vi "Q8381 REF LEVEL_AUTO.vi"(1 "off/on":sgl(ring) items=["OFF", "ON"], 2 "GPIB Sddress":u16=8 max=31 step=1, 3 "VISA resource name":refnum<visa-resource-name>) -> (0 "GPIB Status":bool)   [LabVIEW 2017]
doc: "off/on: 0: off, 1: on."
panel:
  out "Program Code":string
  # "REF  LEVEL__AUTO"
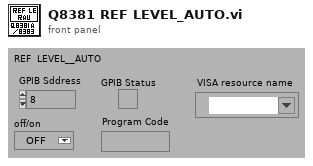
[diagram p1: front panel]
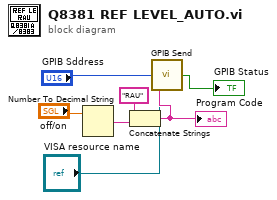
[diagram p0: block diagram]
diagram:
  n1 = Number To Decimal String(number="off/on") -> (decimal integer string=w5:string)  [unwired: 1 in]
  n2 = Concatenate Strings("RAU", w5) -> (w3:string)
  "Program Code" <- w3
  n3 = call "GPIB Send.vi"("Command String"=w3, "Address"="GPIB Sddress", "VISA resource name"="VISA resource name") -> ("Error"=→"GPIB Status":bool)
